vi "Main_Run.vi"() -> ()   [LabVIEW 2019, in "Motor_Lib.lvlib"]
uses:
  Motor_Lib.lvlib
  <vilib>/Platform/TimedLoop/XDataNode/timing_clust.ctl
  <vilib>/Platform/TimedLoop/XDataNode/nitl_modes.ctl
  <vilib>/Platform/TimedLoop/XDataNode/wakeup.ctl
  PORT_ID.ctl
  MotorType.ctl
  <vilib>/myRIO/Common/Instrument Driver Framework/myRIO v1.0/UART/vis/myRIO v1.0 Close UART.vi
  <vilib>/myRIO/Common/Instrument Driver Framework/Utilities/vis/FPGA Ref Manager.vi
  <vilib>/myRIO/Common/Instrument Driver Framework/myRIO v1.0/myRIO v1.0 Reset FPGA.vi
  <vilib>/myRIO/Common/Instrument Driver Framework/myRIO v1.0/IRQ/vis/myRIO v1.0 IRQ Info FGV.vi
  <vilib>/myRIO/Common/Instrument Driver Framework/myRIO v1.0/IRQ/vis/myRIO v1.0 Timer IRQ Info FGV.vi
  <vilib>/myRIO/Common/Instrument Driver Framework/myRIO v1.0/IRQ/vis/myRIO v1.0 ISR Agent.vi
  <vilib>/myRIO/Instrument Drivers/Utilities/vis/Reset Index.vi
  <vilib>/myRIO/Common/Instrument Driver Framework/myRIO v1.0/Resource Manager/vis/myRIO v1.0 Block Write Resource Manager.vi
  <vilib>/platform/TimedLoop/XDataNode/XDataNode.xnode
  <vilib>/Platform/TimedLoop/XDataNode/XDNodeRunTimeDep.lvlib
  <vilib>/myRIO/Instrument Drivers/Utilities/Utilities.lvlib
panel:
  out "Finished Late? [i-1]":bool
  in  "ResetB":bool
  out "RPM/T Chart(Motor B)":T1(graph)
  out "RPM/T Chart(Motor A)":cluster{"upper limit":dbl, "RPM":dbl}(graph)
  out "error out":errorcluster
  in  "TargetRPM(Motor B)":dbl format="%.2f"
  in  "TargetRPM(Motor A)":dbl format="%.2f"
  in  "ResetA":bool
  in  "stop":bool
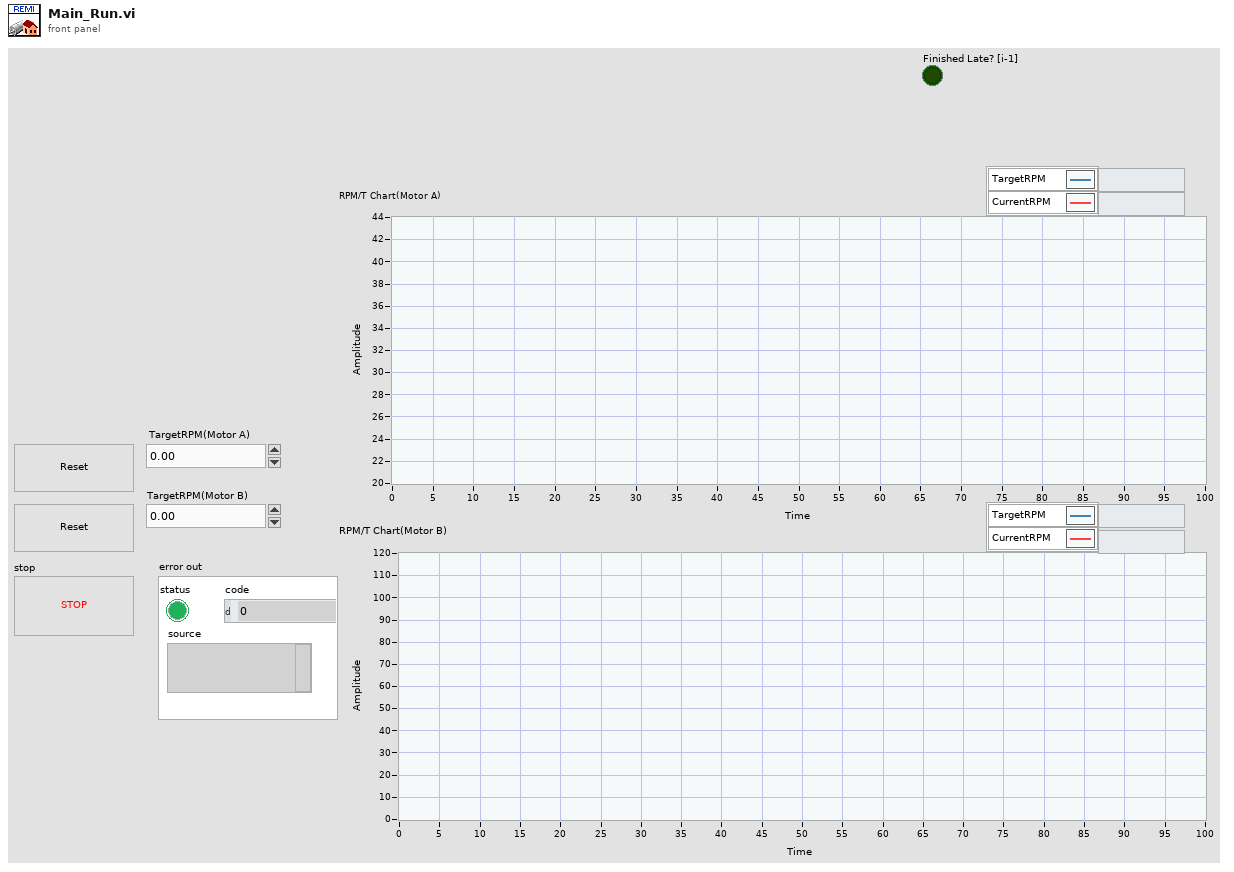
[diagram p1: front panel]
types:
  T1 = cluster{"TargetRPM(Motor B)":dbl, "Rotations":dbl}
  T2 = typedef "MotorType.ctl" = u16
  T3 = typedef "PORT_ID.ctl" = enum16{"PORT_A", "PORT_B"}
  T4 = typedef "XDNodeRunTimeDep.lvlib/timing_clust.ctl" = cluster{"Expected End [f-1]":u64, "Actual End [f-1]":u64, "Finished Late? [f-1]":bool, "Expected End [i-1]":u64, "Actual End [i-1]":u64, "Finished Late? [i-1]":bool, "Expected Start [i]":u64, "Actual Start [i]":u64, "Expected Start [f]":u64, "Actual Start [f]":u64, "Source Name":string, "Structure Name":string, "Period":i64, "Deadline":i64, "Offset":i64, "Start":i64, "Priority":i32, "Timeout":i32, "Mode":T5, "Wakeup Reason":T6, "Error":errorcluster, "Source Type":string, "Secondary Source Type":string, "Global End Time":u64, "Global Start Time":u64, "Frame Duration":u64, "Iteration Duration":u64, "Assigned CPU":i32, "I/O Scan Engine Mode":u32}
  T5 = typedef "XDNodeRunTimeDep.lvlib/nitl_modes.ctl" = enum32{"No Change", "Process missed periods, maintain original phase", "Discard missed periods, maintain original phase", "Process missed periods, ignore original phase", "Discard missed periods, ignore original phase"}
  T6 = typedef "XDNodeRunTimeDep.lvlib/wakeup.ctl" = enum32{"Normal", "Aborted", "Asynchronous wakeup", "Timing source error", "Timed loop error", "Timeout"}
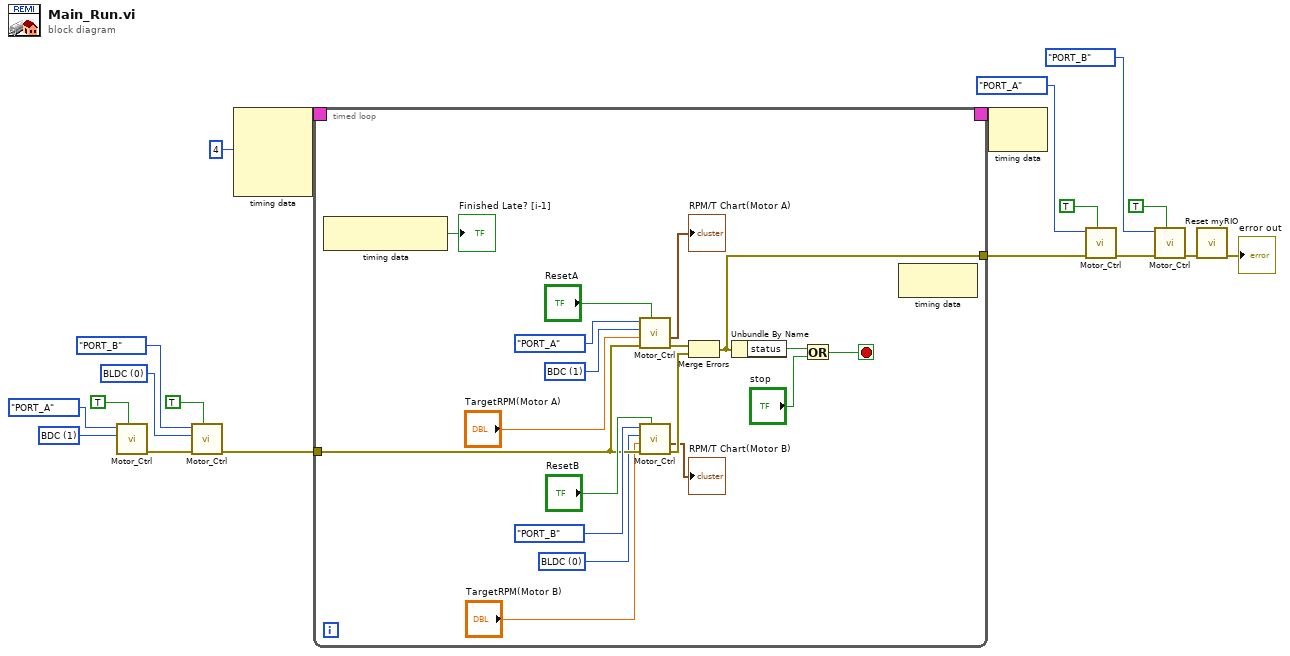
[diagram p0: block diagram]
diagram:
  w1 = T2 0 items=["BLDC", "BDC"] ("B/BL Motor")
  w2 = T2 1 items=["BLDC", "BDC"] ("B/BL Motor")
  n1 = call "Motor_Ctrl.vi"("Reset"=TRUE, "B/BL Motor"=w2, "Port"=PORT_ID."PORT_A") -> ("error out"=w4:errorcluster)  [unwired: 5 in, 3 out]
  n2 = call "Motor_Ctrl.vi"("Reset"=TRUE, "error in (no error)"=w4, "B/BL Motor"=w1, "Port"=PORT_ID."PORT_B") -> ("error out"=w3:errorcluster)  [unwired: 4 in, 3 out]
  n3 = node-c288(i64 4 ("Period")) -> (w19:T4)  [unwired: 3 in]
  n4 = timed-loop {
    timing: w19 -> [_]
    timing-out: [_] -> w18
    tunnel: [w32] -> w11
    tunnel: w3 -> [w26]
    stop <- w29 stop-if-true
    w23 = T2 1 items=["BLDC", "BDC"] ("B/BL Motor")
    w25 = T2 0 items=["BLDC", "BDC"] ("B/BL Motor")
    n5 = node-c288() -> (→"Finished Late? [i-1]":bool)  [unwired: 1 in]
    n6 = call "Motor_Ctrl.vi"("Reset"="ResetA", "error in (no error)"=w26, "TargetRPM(+/-120)"="TargetRPM(Motor A)", "B/BL Motor"=w23, "Port"=PORT_ID."PORT_A" ("PORT")) -> ("error out"=w34:errorcluster, "RPM/T Chart"=→"RPM/T Chart(Motor A)":cluster{"upper limit":dbl, "RPM":dbl})  [unwired: 3 in, 2 out]
    n7 = call "Motor_Ctrl.vi"("Reset"="ResetB", "error in (no error)"=w26, "TargetRPM(+/-120)"="TargetRPM(Motor B)", "B/BL Motor"=w25, "Port"=PORT_ID."PORT_B" ("PORT")) -> ("error out"=w33:errorcluster, "RPM/T Chart"=→"RPM/T Chart(Motor B)":cluster{"upper limit":dbl, "RPM":dbl})  [unwired: 3 in, 2 out]
    n8 = Merge Errors(w34, w33) -> (w32:errorcluster)
    n9 = Unbundle By Name(w32) -> ("status"=w30:bool)
    n10 = Or(x=w30, y="stop") -> (x .or. y?=w29:bool)
    n11 = node-c288() -> ()  [unwired: 1 in, 1 out]
  }
  n12 = node-c288(w18) -> ()  [unwired: 1 out]
  n13 = call "Motor_Ctrl.vi"("Reset"=TRUE, "error in (no error)"=w11, "Port"=PORT_ID."PORT_A") -> ("error out"=w12:errorcluster)  [unwired: 5 in, 3 out]
  n14 = call "Motor_Ctrl.vi"("Reset"=TRUE, "error in (no error)"=w12, "Port"=PORT_ID."PORT_B") -> ("error out"=w10:errorcluster)  [unwired: 5 in, 3 out]
  n15 = call <vilib>:"Reset myRIO.vi"("error in (no error)"=w10) -> ("error out"=→"error out":errorcluster)  [unwired: 10 in]
